vi "Write ArgumentKw Payload.vi"(8 "error in (no error)":errorcluster, 10 "ArgumentKw Payload":string="{}", 11 "CallResult JSON in":refnum<class "CallResult JSON.lvclass">) -> (0 "error out":errorcluster, 3 "CallResult JSON out":refnum<class "CallResult JSON.lvclass">)   [LabVIEW 2020, in "wamplv.lvlib" / "CallResult JSON.lvclass"]
uses:
  CallResult JSON.lvclass
  CallResult JSON.lvclass/CallResult JSON.ctl
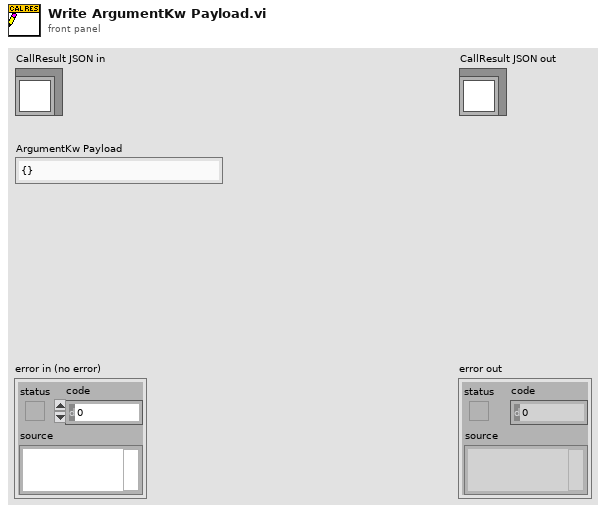
[diagram p1: front panel]
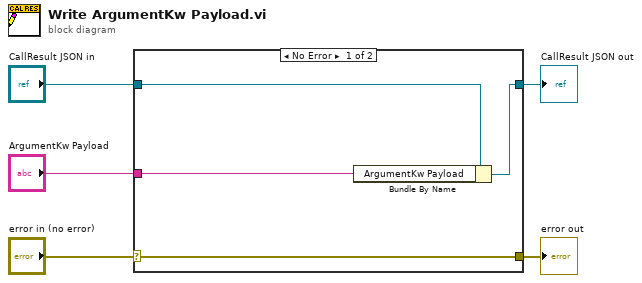
[diagram p0: block diagram]
diagram:
  n1 = case shown="No Error" "error in (no error)" {
    selector: "error in (no error)" -> [w9 w10]
    tunnel: [w9 w10] -> w4
    tunnel: [w7 w11] -> w2
    tunnel: "CallResult JSON in" -> [w8 w11]
    tunnel: "ArgumentKw Payload" -> [w6 _]
    frame No Error {
      n2 = Bundle By Name(cluster=w8, "ArgumentKw Payload"=w6) -> (w7:refnum<class "CallResult JSON.lvclass">)
    }
    frame Error {
    }
  }
  "error out" <- w4
  "CallResult JSON out" <- w2
